vi "Scheduler.FireEvent.vi"(8 "error in":errorcluster, 11 "Sched Item":T1) -> (0 "error out":errorcluster, 3 "Sched Item Out":T1)   [LabVIEW 2024, in "EQMF.lvlib" / "Scheduler.lvlib"]
uses:
  Scheduler.lvlib
  Scheduler.Item.ctl
  Queues/Q.Element.ctl
  Queues/Queue Utils.lvlib
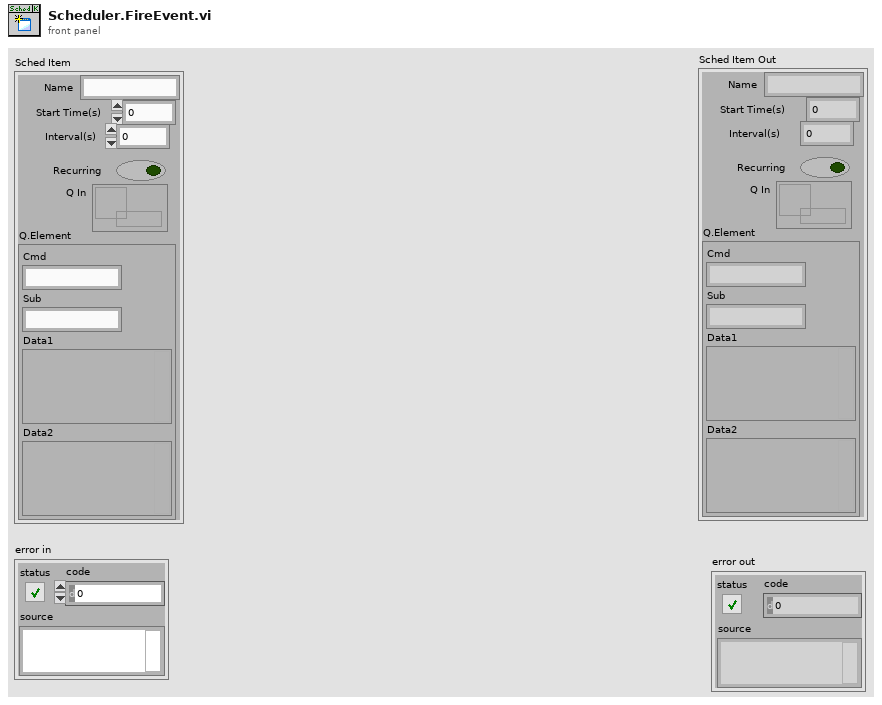
[diagram p1: front panel]
types:
  T1 = typedef "EQMF.lvlib/Scheduler.lvlib/Scheduler.Item.ctl" = cluster{"Name":string, "Start Time(s)":dbl, "Interval(s)":dbl, "Recurring":bool, "Q In":refnum<queue>, "Q.Element":T2}
  T2 = typedef "EQMF.lvlib/Queue Utils.lvlib/Q.Element.ctl" = cluster{"Cmd":string, "Sub":string, "Data1":variant, "Data2":variant}
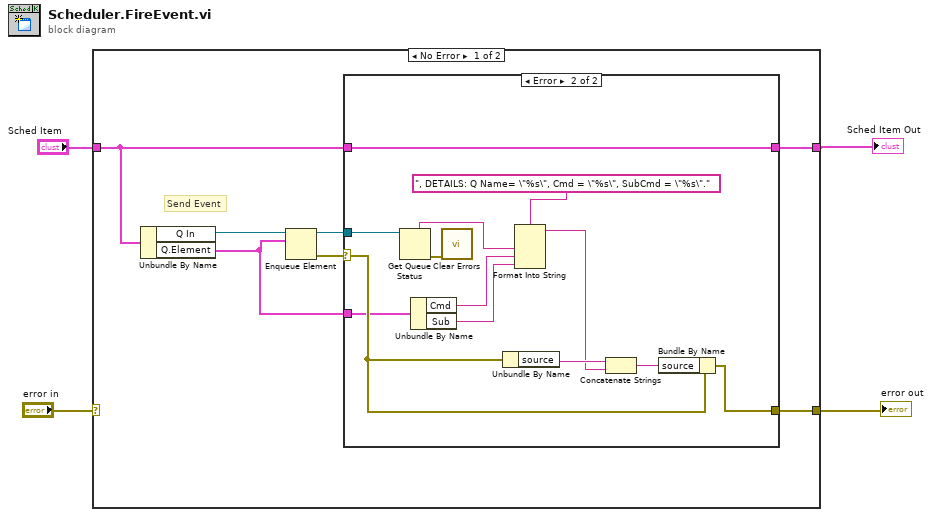
[diagram p0: block diagram]
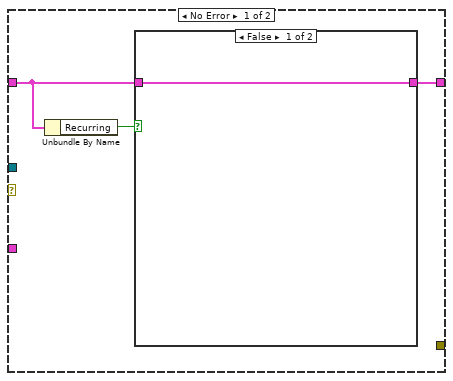
[diagram p2: hidden frame]
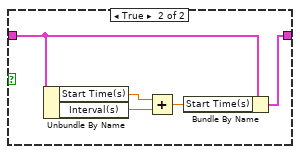
[diagram p3: hidden frame]
diagram:
  n1 = case shown="No Error" "error in" {
    selector: "error in" -> [_ w35]
    tunnel: "Sched Item" -> [w10 w34]
    tunnel: [w9 w34] -> w2
    tunnel: [w8 w35] -> w1
    frame No Error {
      # "Send Event"
      n2 = Unbundle By Name(w10) -> ("Q In"=w7:refnum<queue>, "Q.Element"=w6:T2)
      n3 = Enqueue Element(queue=w7, element=w6) -> (queue out=w5:refnum<queue>, error out=w11:errorcluster)  [unwired: 2 in, 1 out]
      n4 = case shown="Error" w11 {
        selector: w11 -> [_ w29]
        tunnel: w10 -> [w13 w33]
        tunnel: [w12 w33] -> w9
        tunnel: [_ w30] -> w8
        tunnel: w6 -> [_ w26]
        tunnel: w5 -> [_ w32]
        frame No Error {
          n5 = Unbundle By Name(w13) -> ("Recurring"=w14:bool)
          n6 = case shown="False" w14 {
            tunnel: w13 -> [w15 w17]
            tunnel: [w15 w16] -> w12
            frame False {
            }
            frame True {
              n7 = Unbundle By Name(w17) -> ("Start Time(s)"=w20:dbl, "Interval(s)"=w19:dbl)
              n8 = Add(x=w20, y=w19) -> (x+y=w18:dbl)
              n9 = Bundle By Name(cluster=w17, "Start Time(s)"=w18) -> (w16:T1)
            }
          }
        }
        frame Error {
          n10 = Get Queue Status(queue=w32) -> (queue name=w25:string, error out=w21:errorcluster)  [unwired: 2 in, 6 out]
          n11 = Unbundle By Name(w26) -> ("Cmd"=w24:string, "Sub"=w23:string)
          n12 = call <vilib>:"Clear Errors.vi"("error in (no error)"=w21) -> ()  [unwired: 5 in, 2 out]
          n13 = Unbundle By Name(w29) -> ("source"=w28:string)
          n14 = Format Into String(format string=", DETAILS: Q Name= \"%s\", Cmd = \"%s\", SubCmd = \"%s\".", w25, w24, w23) -> (resulting string=w27:string)  [unwired: 2 in, 1 out]
          n15 = Concatenate Strings(w28, w27) -> (w22:string)
          n16 = Bundle By Name(cluster=w29, "source"=w22) -> (w30:errorcluster)
        }
      }
    }
    frame Error {
    }
  }
  "error out" <- w1
  "Sched Item Out" <- w2
